vi "driveToCreateCommands.vi"(8 "toFreestyle":bool, 9 "toDriveDistance":bool, 10 "toTurnAngle":bool, 11 "toDoNothing":bool) -> (3 "Current state":T1)   [LabVIEW 2017]
uses:
  Drive Logic/driveLogicStates.ctl
  <vilib>/FRCT Team# 3937  Breakaway/Memory Library/memLib.lvlib
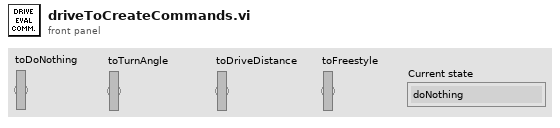
[diagram p1: front panel]
types:
  T1 = typedef "driveLogicStates.ctl" = enum16{"doNothing", "driveDistance", "turnAngle", "freestyle", "guidedDrive", "approachingElement"}
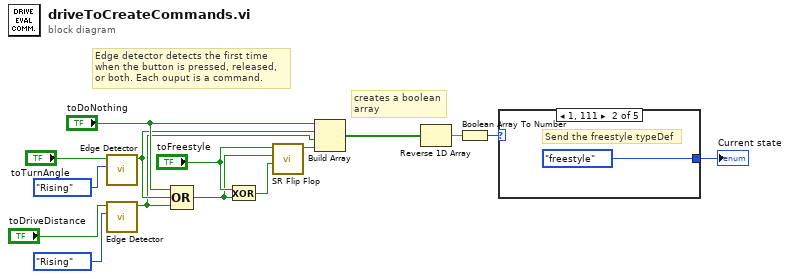
[diagram p0: block diagram]
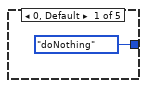
[diagram p2: hidden frame]
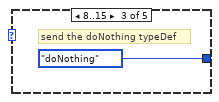
[diagram p3: hidden frame]
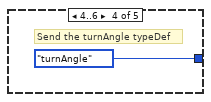
[diagram p4: hidden frame]
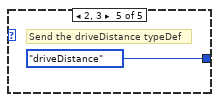
[diagram p5: hidden frame]
diagram:
  # "Edge detector detects the first time\nwhen the button is pressed, released,\nor both. Each ouput is a command."
  # "creates a boolean\narray"
  n1 = call <vilib>:"Edge Detector.vi"("Mode"=enum16{"Rising", "Falling", "Any"}."Rising", "Input"="toTurnAngle") -> ("Output"=w6:bool)  [unwired: 9 in]
  n2 = call <vilib>:"Edge Detector.vi"("Mode"=enum16{"Rising", "Falling", "Any"}."Rising", "Input"="toDriveDistance") -> ("Output"=w1:bool)  [unwired: 9 in]
  n3 = Compound Arithmetic op=OR("toDoNothing", w6, w1) -> (w4:bool)
  n4 = Exclusive Or(1:w4, 2:"toFreestyle") -> (0:w3:bool)
  n5 = call <vilib>:"SR Flip Flop.vi"("Enable"=w3, "Reset"=w4, "Set"="toFreestyle") -> ("Output"=w8:bool)  [unwired: 8 in]
  n6 = Build Array("toDoNothing", w6, w1, w8) -> (w13:bool[])
  n7 = Reverse 1D Array(array=w13) -> (reversed array=w12:bool[])
  n8 = Boolean Array To Number(Boolean array=w12) -> (number=w14:u32)
  n9 = case shown="1, 111" w14 {
    tunnel: [driveLogicStates."doNothing" driveLogicStates."freestyle" driveLogicStates."doNothing" driveLogicStates."turnAngle" driveLogicStates."driveDistance"] -> w15
    frame 0, Default {
    }
    frame 1, 7 {
      # "Send the freestyle typeDef"
    }
    frame 8..15 {
      # "send the doNothing typeDef"
    }
    frame 4..6 {
      # "Send the turnAngle typeDef"
    }
    frame 2, 3 {
      # "Send the driveDistance typeDef"
    }
  }
  "Current state" <- w15
